vi "Initialize Hardware References Piezo.vi"(8 "error in (no error)":errorcluster, 11 "Hardware Configuration":T1) -> (0 "error out":errorcluster, 3 "Hardware Configuration 2":T1)   [LabVIEW 2013]
uses:
  Hardware Configuration Piezo.ctl
  Piezo/Piezo.lvlib
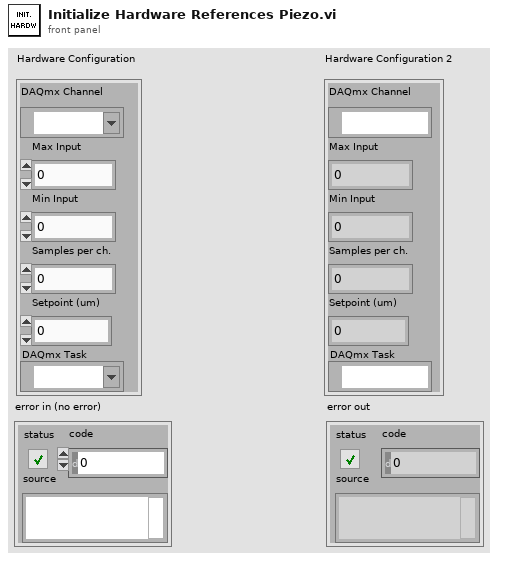
[diagram p1: front panel]
types:
  T1 = typedef "Piezo.lvlib/Hardware Configuration Piezo.ctl" = cluster{"DAQmx Channel":tag, "Max Input":dbl, "Min Input":dbl, "Samples per ch.":dbl, "Setpoint (um)":dbl, "DAQmx Task":refnum<k21>}
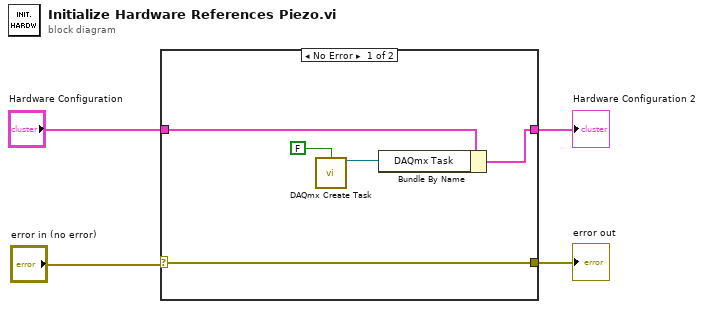
[diagram p0: block diagram]
diagram:
  n1 = case shown="No Error" "error in (no error)" {
    selector: "error in (no error)" -> [w9 w11]
    tunnel: [w9 w11] -> w3
    tunnel: "Hardware Configuration" -> [w7 w10]
    tunnel: [w5 w10] -> w1
    frame No Error {
      n2 = call <vilib>:"DAQmx Create Task.vi"("auto cleanup"=FALSE) -> ("task out"=w6:refnum<k21>)  [unwired: 13 in, 1 out]
      n3 = Bundle By Name(cluster=w7, "DAQmx Task"=w6) -> (w5:T1)
    }
    frame Error {
    }
  }
  "Hardware Configuration 2" <- w1
  "error out" <- w3
